vi "Init Control.vi"(5 "Group":refnum<class "Group DBL.lvclass">, 6 "Period ms":i64, 7 "VolatusAPI":refnum<class "VolatusAPI.lvclass">, 8 "error in (no error)":errorcluster, 9 "Control MsgQ":refnum<class "MessageQ.lvclass">, 10 "Config Element":refnum<class "Config Element.lvclass">, 11 "Valve in":refnum<class "DigitalControl.lvclass">) -> (0 "error out":errorcluster, 3 "Valve out":refnum<class "DigitalControl.lvclass">)   [LabVIEW 2020, in "VolatusControl.lvlib" / "DigitalControl.lvclass"]
uses:
  DigitalControl.lvclass
  lv-cdm/CDM-Config/Config Element/Config Element.lvclass
  Volatus/VolatusAPI/VolatusAPI.lvclass
  Volatus/MessageQ/MessageQ.lvclass
  lv-vecto/Vecto/Group DBL/Group DBL.lvclass
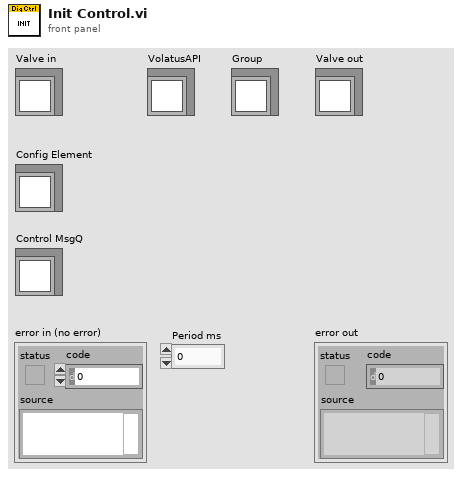
[diagram p1: front panel]
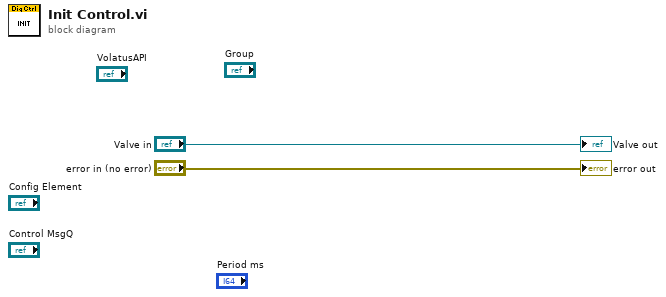
[diagram p0: block diagram]
diagram:
  "error out" <- "error in (no error)"
  "Valve out" <- "Valve in"
